vi "WriteText.vi"(1 "filename":string, 2 "Input data":string[][](array[string]), 3 "Append":bool, 4 "httpRequestID":u32) -> (0 "hyperlink":string)   [LabVIEW 2011]
uses:
  <vilib>/Utility/file.llb/Write To Spreadsheet File (string).vi
  <vilib>/wsapi/NI_WebServices.lvlib
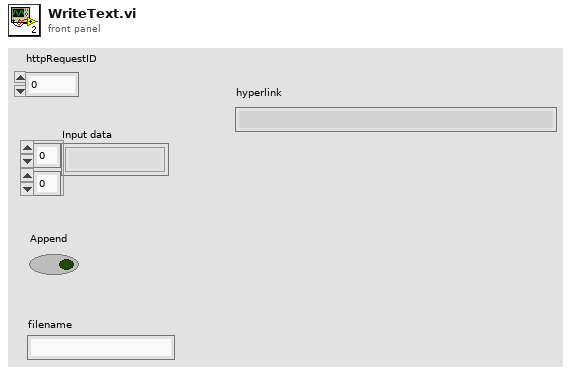
[diagram p1: front panel]
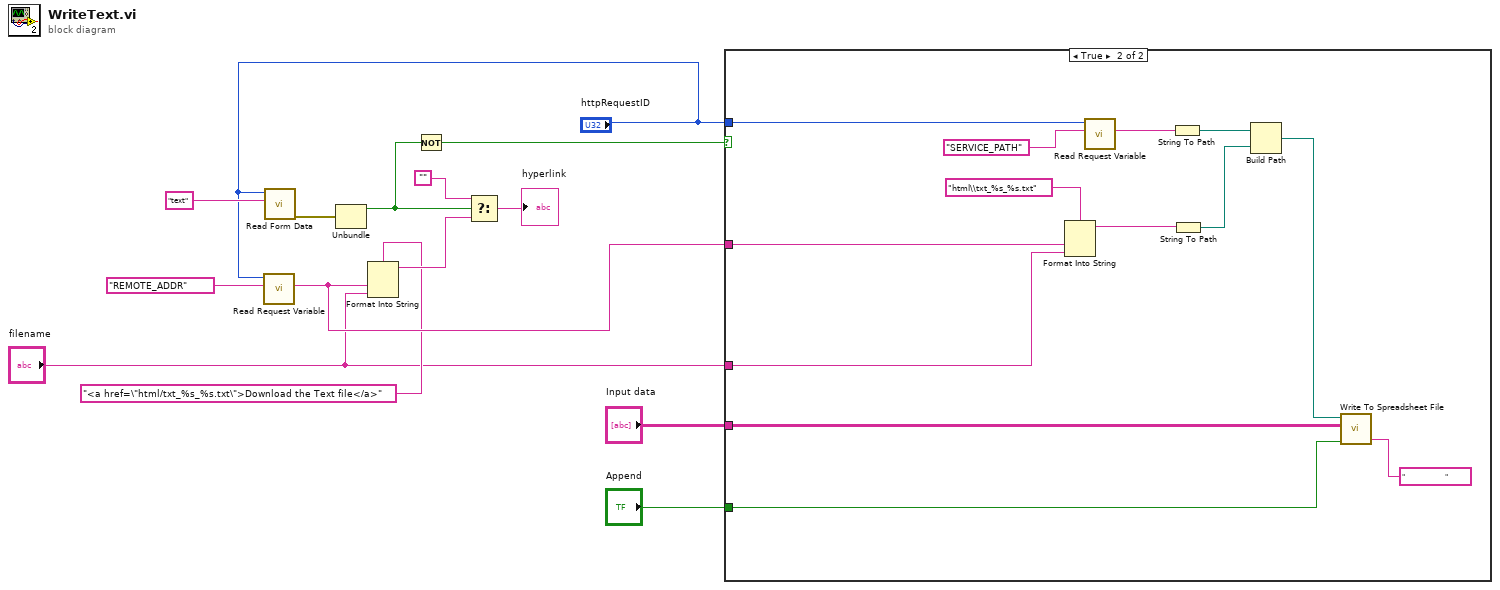
[diagram p0: block diagram]
diagram:
  n1 = call <vilib>:"Read Request Variable.vi"("variable name"="REMOTE_ADDR", "httpRequestID"="httpRequestID") -> ("value"=w3:string)  [unwired: 7 in, 2 out]
  n2 = call <vilib>:"Read Form Data.vi"("key"="text", "httpRequestID"="httpRequestID") -> ("error out"=w12:errorcluster)  [unwired: 1 in, 8 out]
  n3 = Unbundle(w12) -> ("status"=w10:bool)  [unwired: 2 out]
  n4 = Format Into String(format string="<a href=\"html/txt_%s_%s.txt\">Download the Text file</a>", w3, "filename") -> (resulting string=w8:string)  [unwired: 2 in, 1 out]
  n5 = Not(x=w10) -> (.not. x?=w6:bool)
  n6 = Select(t="", s=w10, f=w8) -> (s? t:f=→"hyperlink":string)
  n7 = case shown="True" w6 {
    tunnel: "Input data" -> [_ w21]
    tunnel: "httpRequestID" -> [_ w20]
    tunnel: "Append" -> [_ w19]
    tunnel: w3 -> [_ w16]
    tunnel: "filename" -> [_ w15]
    frame False {
    }
    frame True {
      n8 = Format Into String(format string="html\\txt_%s_%s.txt", w16, w15) -> (resulting string=w17:string)  [unwired: 2 in, 1 out]
      n9 = call <vilib>:"Read Request Variable.vi"("variable name"="SERVICE_PATH", "httpRequestID"=w20) -> ("value"=w26:string)  [unwired: 7 in, 2 out]
      n10 = String To Path(string=w26) -> (path=w25:path)
      n11 = String To Path(string=w17) -> (path=w23:path)
      n12 = Build Path(base path=w25, name or relative path=w23) -> (appended path=w22:path)
      n13 = call-poly <vilib>:"Write To Spreadsheet File.vi"("delimiter (\\t)"="                    ", "append to file? (new file:F)"=w19, "2D data"=w21, "file path (dialog if empty)"=w22) -> ()  [unwired: 4 in, 1 out]
    }
  }
